vi "RunTest.vi"(8 "error in (no error)":errorcluster, 11 "TestCaseMock in":refnum<class "TestCaseMock.lvclass">) -> (0 "error out":errorcluster, 3 "TestCaseMock out":refnum<class "TestCaseMock.lvclass">)   [LabVIEW 2019, in "TestResultTestSupport.lvlib" / "TestCaseMock.lvclass"]
doc: "Override to run the test and assert its state."
uses:
  TestCaseMock.lvclass
  TestCaseMock.lvclass/TestCaseMock.ctl
  Error/Error.lvlib
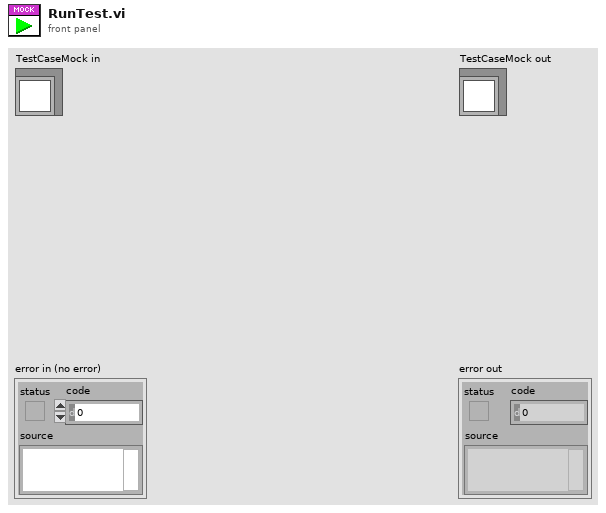
[diagram p1: front panel]
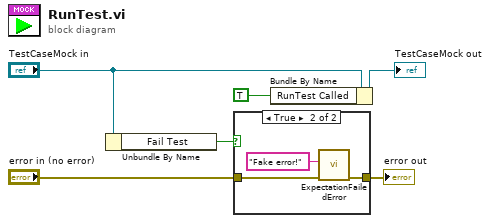
[diagram p0: block diagram]
diagram:
  n1 = Unbundle By Name("TestCaseMock in") -> ("Fail Test"=w1:bool)
  n2 = case shown="True" w1 {
    tunnel: "error in (no error)" -> [w7 w9]
    tunnel: [w7 w10] -> w2
    frame False {
    }
    frame True {
      n3 = call "ExpectationFailedError.vi"("error in (no error)"=w9, "Message"="Fake error!") -> ("error out"=w10:errorcluster)  [unwired: 9 in]
    }
  }
  "error out" <- w2
  n4 = Bundle By Name(cluster="TestCaseMock in", "RunTest Called"=TRUE ("RunBare Called")) -> (→"TestCaseMock out":refnum<class "TestCaseMock.lvclass">)
